vi "Create Event.vi"(9 "Event":refnum<class "Event.lvclass">, 10 "Self Event Alias":string, 11 "Template Queue in":refnum<class "Template Queue.lvclass">) -> (3 "Template Queue out":refnum<class "Template Queue.lvclass">)   [LabVIEW 2021, in "Template Queue.lvlib" / "Template Queue.lvclass"]
uses:
  Template Queue.lvclass
  <vilib>/Nathan Davis/jettl/jettl/Event/Event.lvclass
  Template Queue.lvclass/Template Queue.ctl
  <vilib>/Nathan Davis/jettl/jettl/Queue/Queue.lvclass
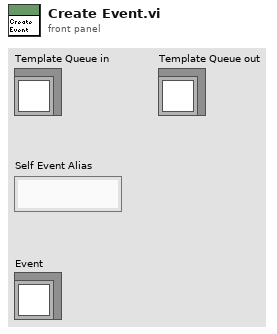
[diagram p1: front panel]
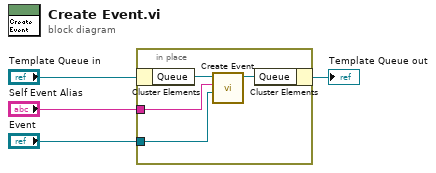
[diagram p0: block diagram]
diagram:
  n1 = in-place {
    in-place-border: "Self Event Alias" -> [w6]
    in-place-border: "Event" -> [w5]
    n2 = in-place-cluster #1("Template Queue in") -> ("Queue"=w8:refnum<class "Queue.lvclass">)
    n3 = call-dynamic "Create Event.vi"("Event"=w5, "Self Event Alias"=w6, "jettl Msg Create Event in"=w8) -> ("jettl Msg Create Event out"=w7:refnum<class "Queue.lvclass">)  [unwired: 8 in]
    n4 = in-place-cluster #1("Queue"=w7) -> (→"Template Queue out":refnum<class "Template Queue.lvclass">)
  }
